vi "FrameID to Frame Ref.vi"(7 "Database alias":string="Database", 8 "error in (no error)":errorcluster, 11 "Frame ID":u32) -> (0 "error out":errorcluster, 2 "Found":bool, 3 "Frame Name":refnum<k21>)   [LabVIEW 2021]
uses:
  <resource>/objmgr/xnet.rc
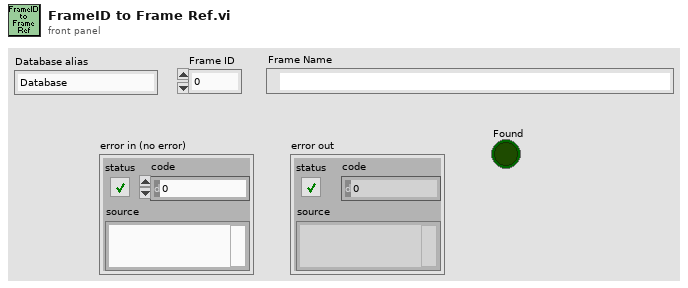
[diagram p1: front panel]
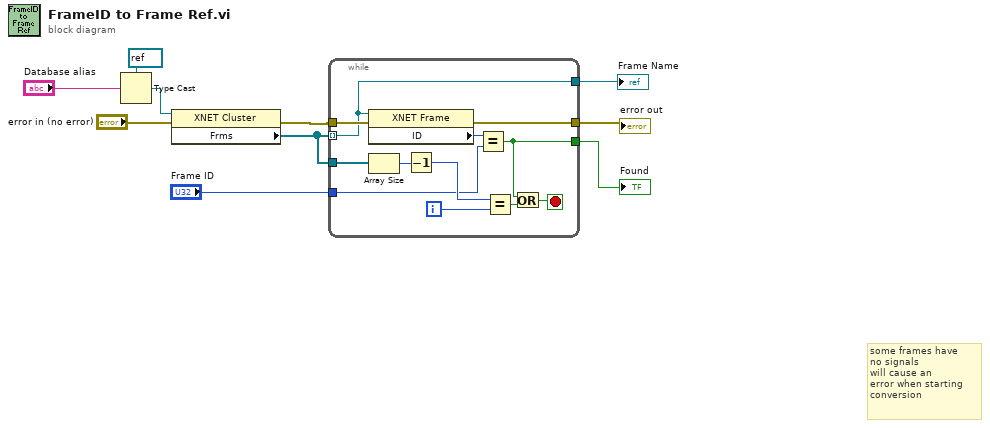
[diagram p0: block diagram]
diagram:
  # "some frames have\nno signals\nwill cause an \nerror when starting\nconversion"
  n1 = Type Cast(type=refnum<k21> refnum ("cluster (:memory:)"), x="Database alias") -> (*(type *) &x=w5:refnum<k21>)
  n2 = property class="XNET Cluster"(reference=w5, error in="error in (no error)") -> (error out=w9:errorcluster, "Frms"=w10:refnum<k21>[])  [unwired: 1 out]
  n3 = while {
    tunnel: w10 -> [w12] mode=indexing
    tunnel: w9 -> [w22]
    tunnel: w10 -> [w19]
    tunnel: [w12] -> w2
    tunnel: [w16] -> w3
    tunnel: [w15] -> w1
    tunnel: "Frame ID" -> [w11]
    i -> [w13]
    stop <- w20 stop-if-true
    n4 = property class="XNET Frame"(reference=w12, error in=w22) -> (error out=w15:errorcluster, "ID"=w21:u32)  [unwired: 1 out]
    n5 = Array Size(array=w19) -> (size(s)=w18:i32)
    n6 = Decrement(x=w18) -> (x-1=w14:i32)
    n7 = Equal?(x=w21, y=w11) -> (x = y?=w16:bool)
    n8 = Equal?(x=w14, y=w13) -> (x = y?=w17:bool)
    n9 = Or(x=w16, y=w17) -> (x .or. y?=w20:bool)
  }
  "error out" <- w1
  "Frame Name" <- w2
  "Found" <- w3
